vi "Video Stuff v09.vi"() -> ()   [LabVIEW 2009]
uses:
  <vilib>/userDefined/High Color/IMAQdx.ctl
  <vilib>/vision/NI_Vision_Development_Module.lvlib
  <vilib>/vision/driver/NI_Vision_Acquisition_Software.lvlib
panel:
  in  "Y Min":i32=4
  in  "Y Max":i32=22
  in  "X min":i32=4
  in  "X max":i32=22
  in  "Image Type":T1 items=["Grayscale (U8)", "Grayscale (I16)", "Grayscale (SGL)", "Complex (CSG)", "RGB (U32)", "HSL (U32)", "RGB (U64)", "Grayscale (U16)"]
  in  "Desired X Resolution":i32=640
  in  "LineFilterSelect":bool
  out "Hough Intensity Graph":i32[][](graph)
  out "Angle 2":i32
  out "X Intercept 2":i32
  in  "Hough Skip":i32=1
  out "Waypoint":cluster{i32, i32}
  in  "WP_DisplaySize/2":i32
  out "Filter Binary 2":T2(plugin-control)
  in  "Offset scale":dbl=1.51
  in  "Y":i32=1741
  in  "X":i32=777
  out "Real World Coordinates":cluster{"X":sgl, "Y":sgl} {"Y" format="%.2f"; "X" format="%.2f"}
  in  "Interpolation Type":u32(ring)=1 items=["Zero Order", "Bi-Linear", "Quadratic", "Cubic Spline"]
  in  "X Resolution":i32=640
  in  "Filter Select":T3(radio)
  in  "bin 1    bin 2":bool
  in  "Dan    Me":bool=TRUE
  in  "Numeric":i32=21
  out "Occupancy Grid Square Size":dbl
  in  "LIDAR/Wheel Position Offset (in.)":dbl=60.0
  out "\"Obstickles\" y":dbl[](array[numeric])
  out "\"Obstickles\" x":dbl[](array[numeric])
  out "Small":T2(plugin-control)
  in  "Horizontal Resolution of Small Image":i32=50
  out "Super Filter":T2(plugin-control)
  in  "Color Mode":u16(ring) items=["RGB", "HSL", "HSV", "HSI"]
  in  "Blue Range":cluster{"Lower value":i32, "Upper value":i32}={"Lower value"=20, "Upper value"=255}
  in  "Green Range":cluster{"Lower value":i32, "Upper value":i32}={"Lower value"=180, "Upper value"=255}
  in  "Red Range":cluster{"Lower value":i32, "Upper value":i32}={"Lower value"=150, "Upper value"=255}
  in  "stop":bool
  out "trans":T2(plugin-control)
  out "Buffer Number":u32
  out "Live Video":T2(plugin-control)
  in  "Video Modes":i32(listbox)=20
  in  "Camera Name":T4="cam0"
  in  "Calibration File Path":path=path "C:/Documents and Settings/ekolker/My Documents/OGRE/vision/calibrationGridLargeV2.PNG"
  out "Top Image":T2(plugin-control) caption="Calibration Template"
  # "Line Width Paramaters"
  # "Lower:\n   YUV?\n  150, 180, 20\n   RGB?\n  240, 240, 240"
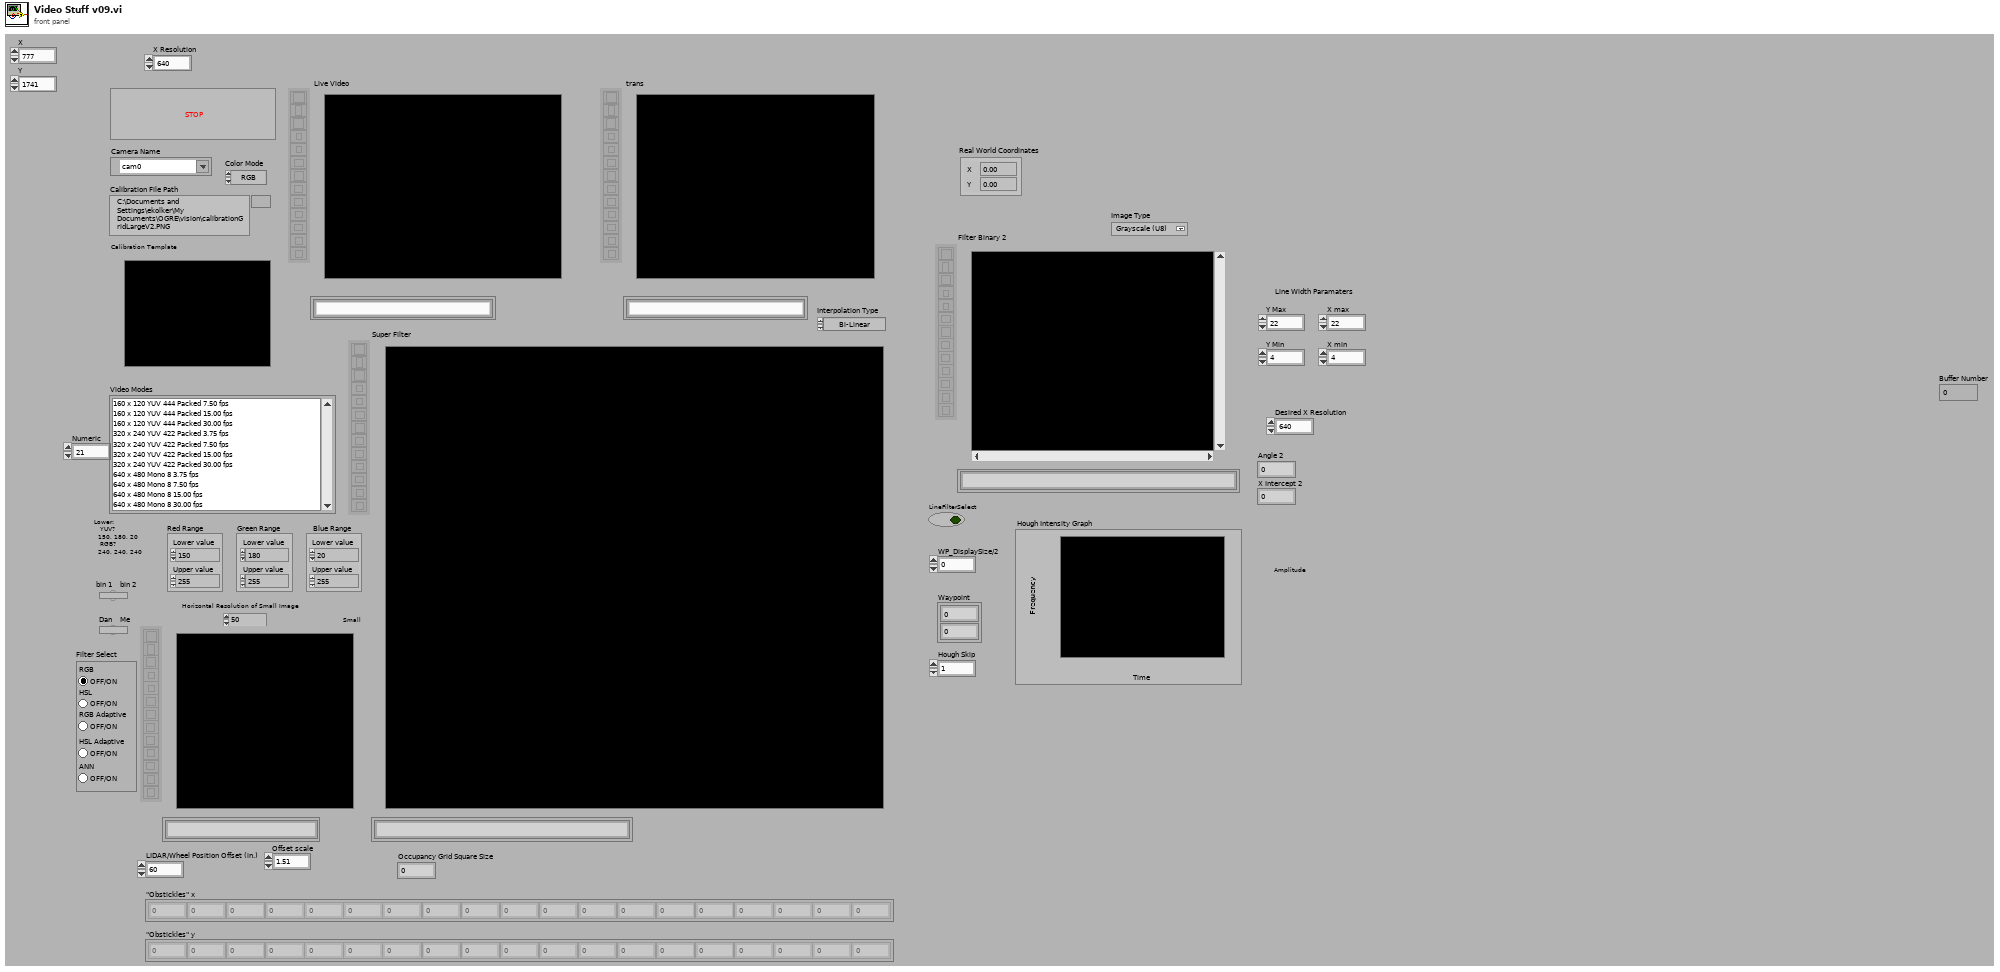
[diagram p1: front panel]
types:
  T1 = typedef "Image Type" = u32
  T2 = typedef "IMAQ Image.ctl" = refnum<image>
  T3 = enum32{"RGB", "HSL", "RGB Adaptive", "HSL Adaptive", "ANN"}
  T4 = typedef "IMAQdx.ctl" = refnum<k21>
  T5 = cluster{"X Step":sgl, "Y Step":sgl, "Unit":u32, "Threshold Range":cluster{"Lower value":sgl, "Upper value":sgl}}
  T6 = cluster{"Distortion":u32, "Corrected Image Scaling":u32, "Corrected Image Learn ROI":u32, "Learn Error Map?":bool, "Learn Correction Table?":bool}
  T7 = cluster{cluster{sgl, sgl}, "Angle Relative to Horizontal (deg)":sgl, "Axis Reference":u32}
  T8 = cluster{"Left":i32, "Top":i32, "Right":i32, "Bottom":i32}
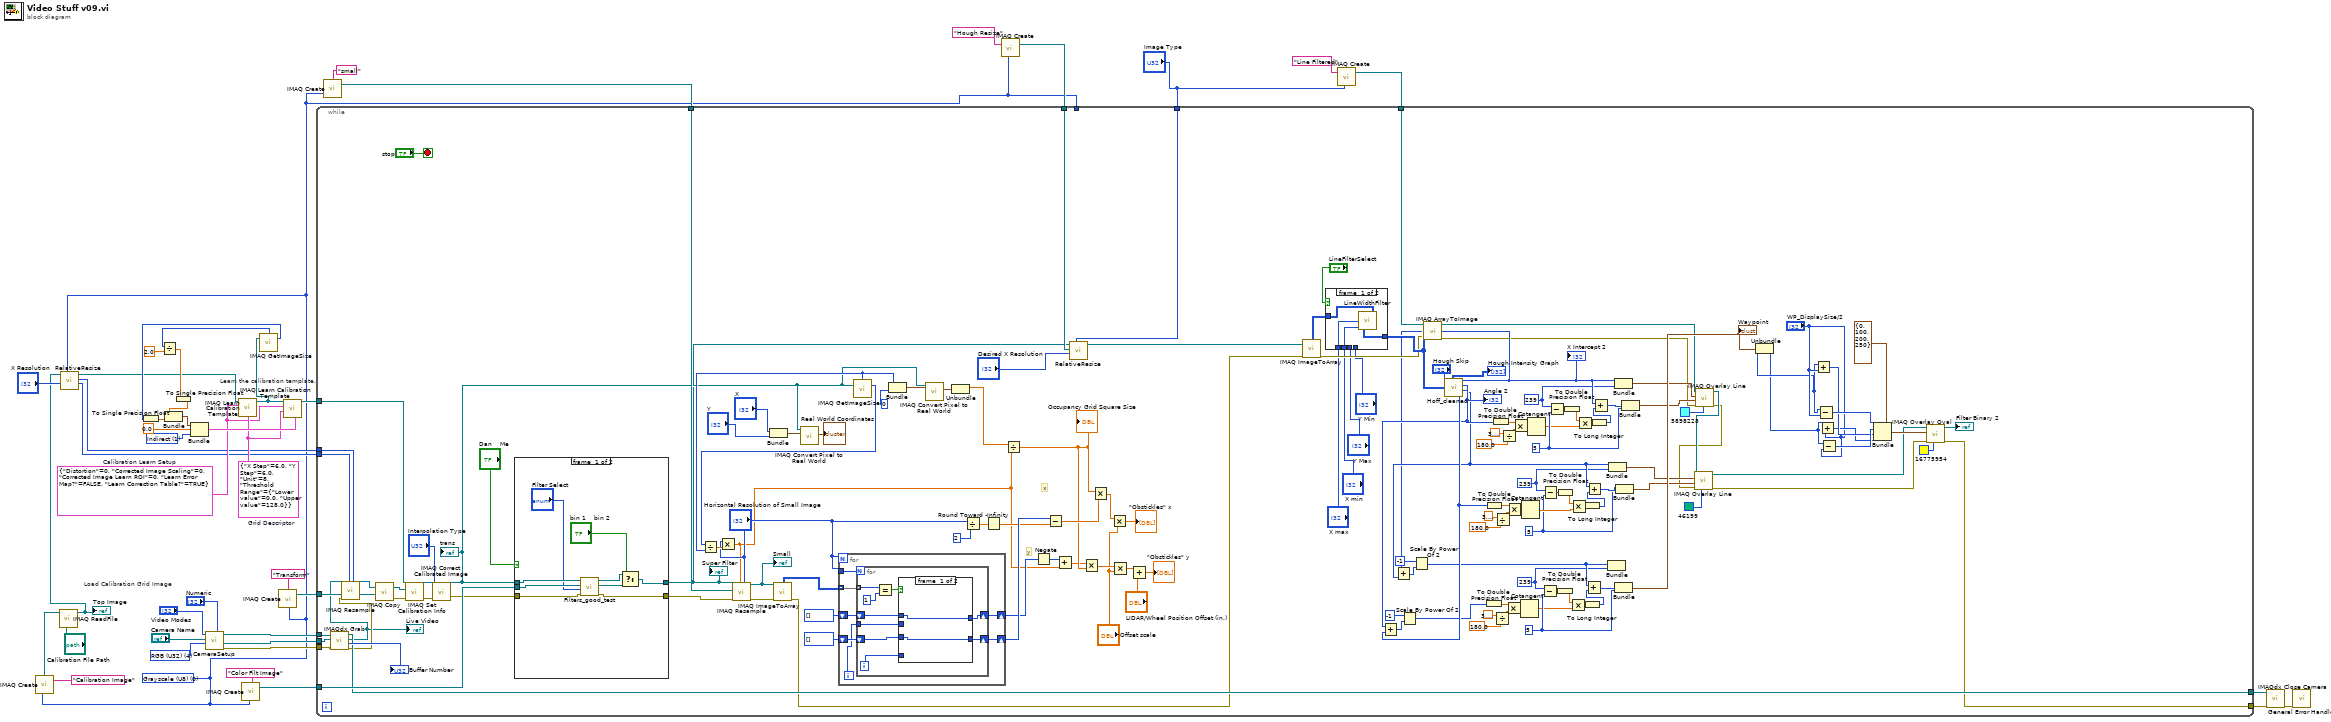
[diagram p0: block diagram]
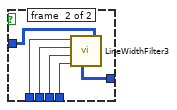
[diagram p2: hidden frame]
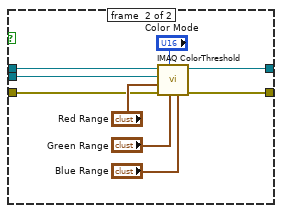
[diagram p3: hidden frame]
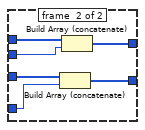
[diagram p4: hidden frame]
diagram:
  w1 = T1 4 items=["Grayscale (U8)", "Grayscale (I16)", "Grayscale (SGL)", "Complex (CSG)", "RGB (U32)", "HSL (U32)", "RGB (U64)", "Grayscale (U16)"] ("Image Type")
  w26 = u32 1 items=["Direct", "Indirect"] ("Axis Reference")
  w3 = T1 0 items=["Grayscale (U8)", "Grayscale (I16)", "Grayscale (SGL)", "Complex (CSG)", "RGB (U32)", "HSL (U32)", "RGB (U64)", "Grayscale (U16)"] ("Image Type")
  w14 = T5 {"X Step"=6.0, "Y Step"=6.0, "Unit"=8, "Threshold Range"={"Lower value"=0.0, "Upper value"=128.0}}  # Grid Descriptor
  w13 = T6 {"Distortion"=0, "Corrected Image Scaling"=0, "Corrected Image Learn ROI"=0, "Learn Error Map?"=FALSE, "Learn Correction Table?"=TRUE}  # Calibration Learn Setup
  # "Load Calibration Grid Image"
  # "Learn the calibration template."
  n1 = call "IMAQ Create"("Image Name"="Calibration Image", "Image Type"=w3) -> ("New Image"=w34:T2)  [unwired: 2 in, 2 out]
  n2 = call "IMAQ ReadFile"("File Path"="Calibration File Path", "Image"=w34) -> ("Image Out"=w8:T2)  [unwired: 3 in, 6 out]
  "Top Image" <- w8
  n3 = call "RelativeResize.vi"("Image Type"=w3, "Desired X Resolution"="X Resolution", "Image"=w8) -> ("Y Resolution"=w6:i32, "X Resolution"=w7:i32, "Image Dst Out"=w9:T2)  [unwired: 3 in, 1 out]
  n4 = call "CameraSetup.vi"("Video Modes"="Video Modes", "Camera Name"="Camera Name", "Image Type"=w1, "Numeric"="Numeric") -> ("Session Out"=w37:T4, "New Image"=w36:T2, "error out"=w35:errorcluster)  [unwired: 2 in]
  n5 = call "IMAQ Learn Calibration Template"("Grid Descriptor"=w14, "Calibration Learn Setup"=w13, "Image"=w9) -> ("Calibrated Image"=w21:T2)  [unwired: 4 in, 4 out]
  n6 = call "IMAQ Create"("Image Name"="Color Filt Image", "Image Type"=w3) -> ("New Image"=w33:T2)  [unwired: 2 in, 2 out]
  n7 = call "IMAQ GetImageSize"("Image"=w21) -> ("Y Resolution"=w18:i32, "X Resolution"=w19:i32)  [unwired: 3 in, 1 out]
  n8 = To Single Precision Float(number=w18) -> (single precision float=w17:sgl)
  n9 = Divide(x=w19, y=2.0) -> (x/y=w16:dbl)
  n10 = To Single Precision Float(number=w16) -> (single precision float=w15:sgl)
  n11 = Bundle(w15, w17) -> (w24:cluster{sgl, sgl})  [unwired: 1 in]
  n12 = Bundle(w24, "Angle Relative to Horizontal (deg)"=sgl 0.0, "Axis Reference"=w26) -> (w22:T7)  [unwired: 1 in]
  n13 = call "IMAQ Create"("Image Name"="Transform", "Image Type"=w3) -> ("New Image"=w38:T2)  [unwired: 2 in, 2 out]
  n14 = call "IMAQ Learn Calibration Template"("Calibration Axis Info"=w22, "Grid Descriptor"=w14, "Calibration Learn Setup"=w13, "Image"=w21) -> ("Calibrated Image"=w23:T2)  [unwired: 3 in, 4 out]
  n15 = call "IMAQ Create"("Image Name"="small", "Image Type"=w3) -> ("New Image"=w31:T2)  [unwired: 2 in, 2 out]
  n16 = call "IMAQ Create"("Image Name"="Hough Resize", "Image Type"=w3) -> ("New Image"=w4:T2)  [unwired: 2 in, 2 out]
  n17 = call "IMAQ Create"("Image Name"="Line Filtered", "Image Type"="Image Type") -> ("New Image"=w11:T2)  [unwired: 2 in, 2 out]
  n18 = while {
    tunnel: w23 -> [w159]
    tunnel: w38 -> [w188]
    tunnel: w37 -> [w187]
    tunnel: w36 -> [w186]
    tunnel: w35 -> [w185]
    tunnel: w33 -> [w181]
    tunnel: w31 -> [w179]
    tunnel: [w177] -> w29
    tunnel: [w120] -> w28
    tunnel: w11 -> [w119]
    tunnel: w7 -> [w59]
    tunnel: w6 -> [w58]
    tunnel: w4 -> [w55]
    tunnel: w3 -> [_]
    tunnel: "Image Type" -> [w54]
    stop <- "stop" stop-if-true
    w104 = 5 ("y")
    w103 = 239 ("y")
    w82 = 5 ("y")
    w83 = 239 ("y")
    w71 = 5 ("y")
    w70 = 239 ("y")
    # "y"
    # "x"
    n19 = call <vilib>:"IMAQdx Grab.vi"("error in"=w185, "Image In"=w186, "Session In"=w187) -> ("error out"=w162:errorcluster, "Buffer Number Out"=→"Buffer Number":u32, "Image Out"=w161:T2, "Session Out"=w177:T4)  [unwired: 1 in, 4 out]
    "Live Video" <- w161
    n20 = call "IMAQ Resample"("X Resolution"=w59, "Y Resolution"=w58, "error in (no error)"=w162, "Image Src"=w161) -> ("Image Dst Out"=w160:T2)  [unwired: 6 in, 1 out]
    n21 = call "IMAQ Copy"("Image Dst"=w188, "Image Src"=w160) -> ("error out"=w189:errorcluster, "Image Dst Out"=w192:T2)  [unwired: 4 in]
    n22 = call "IMAQ Set Calibration Info"("error in (no error)"=w189, "Image Dst"=w192, "Image Src"=w159) -> ("error out"=w190:errorcluster, "Calibrated Image"=w191:T2)  [unwired: 1 in, 6 out]
    n23 = call "IMAQ Correct Calibrated Image"("Interpolation Type"="Interpolation Type", "error in (no error)"=w190, "Image Src"=w191) -> ("error out"=w180:errorcluster, "Corrected Image"=w51:T2)  [unwired: 4 in, 3 out]
    "trans" <- w51
    n24 = case shown="False" "Dan    Me" {
      tunnel: [w211 w217] -> w184
      tunnel: [w208 w216] -> w50
      tunnel: w181 -> [w209 w215]
      tunnel: w180 -> [w212 w214]
      tunnel: w51 -> [w210 w213]
      frame #0 {
        n25 = call "Filters_good_test.vi"("error in"=w212, "Filter Select"="Filter Select", "Filter"=w209, "Input"=w210) -> ("error out"=w211:errorcluster, "Filter Binary"=w207:T2, "Filter Binary 2"=w206:T2)  [unwired: 5 in]
        n26 = Select(t=w206, s="bin 1    bin 2", f=w207) -> (s? t:f=w208:T2)
      }
      frame #1 {
        n27 = call "IMAQ ColorThreshold"("Blue or Luma or Val or Inten Range"="Blue Range", "Green or Sat Range"="Green Range", "Color Mode"="Color Mode", "error in (no error)"=w214, "Red or Hue Range"="Red Range", "Image Dst"=w215, "Image Src"=w213) -> ("error out"=w217:errorcluster, "Image Dst Out"=w216:T2)  [unwired: 3 in]
      }
    }
    "Super Filter" <- w50
    n28 = Bundle("X"="X", "Y"="Y") -> (w155:cluster{"X":i32, "Y":i32})  [unwired: 1 in]
    n29 = call "IMAQ Convert Pixel to Real World"("Pixel Coordinates"=w155, "Calibrated Image"=w51) -> ("Real World Coordinates"=→"Real World Coordinates":cluster{"X":sgl, "Y":sgl})  [unwired: 4 in, 5 out]
    n30 = call "IMAQ GetImageSize"("Image"=w51) -> ("Y Resolution"=w147:i32, "X Resolution"=w146:i32)  [unwired: 3 in, 1 out]
    n31 = Divide(x=w147, y=w146) -> (x/y=w149:dbl)
    n32 = Multiply(x="Horizontal Resolution of Small Image", y=w149) -> (x*y=w140:dbl)
    n33 = call "IMAQ Resample"("X Resolution"="Horizontal Resolution of Small Image", "Y Resolution"=w140, "error in (no error)"=w184, "Image Dst"=w179, "Image Src"=w50) -> ("error out"=w183:errorcluster, "Image Dst Out"=w123:T2)  [unwired: 5 in]
    "Small" <- w123
    n34 = call "IMAQ ImageToArray"("error in (no error)"=w183, "Image"=w123) -> ("error out"=w121:errorcluster, "Image Pixels (U8)"=w174:u8[][])  [unwired: 2 in, 3 out]
    n35 = for {
      N: "Horizontal Resolution of Small Image" -> [_]
      tunnel: "Horizontal Resolution of Small Image" -> [w228]
      tunnel: w174 -> [w227] mode=indexing
      shift-right: [w226] -> w173
      shift-left: i32[] [] -> [w225]
      shift-right: [w223] -> w166
      shift-left: i32[] [] -> [w222]
      i -> [w224]
      n36 = for {
        N: w228 -> [_]
        tunnel: w227 -> [w237] mode=indexing
        shift-right: [w233] -> w226
        shift-left: w225 -> [w232]
        tunnel: w224 -> [w231]
        shift-right: [w230] -> w223
        shift-left: w222 -> [w229]
        i -> [w235]
        n37 = Equal?(x=w237, y=u8 1) -> (x = y?=w234:bool)
        n38 = case shown="False" w234 {
          tunnel: w235 -> [_ w245]
          tunnel: [w238 w244] -> w233
          tunnel: w232 -> [w238 w243]
          tunnel: w231 -> [_ w242]
          tunnel: [w239 w241] -> w230
          tunnel: w229 -> [w239 w240]
          frame #0 {
          }
          frame #1 {
            n39 = Build Array (concatenate)(w243, w245) -> (w244:i32[])
            n40 = Build Array (concatenate)(w240, w242) -> (w241:i32[])
          }
        }
      }
    }
    n41 = Bundle("X Resolution"=w146, 0) -> (w157:cluster{"X Resolution":i32, i32})  [unwired: 1 in]
    n42 = call "IMAQ Convert Pixel to Real World"("Pixel Coordinates"=w157, "Calibrated Image"=w51) -> ("Real World Coordinates"=w151:cluster{"X":sgl, "Y":sgl})  [unwired: 4 in, 5 out]
    n43 = Unbundle(w151) -> ("X"=w150:sgl)  [unwired: 1 out]
    n44 = Divide(x="Horizontal Resolution of Small Image", y=2) -> (x/y=w165:dbl)
    n45 = Round Toward -Infinity(1:w165) -> (0:w164:dbl)
    n46 = Divide(x=w150, y=w140) -> (x/y=w171:dbl)
    "Occupancy Grid Square Size" <- w171
    n47 = Negate(x=w166) -> (-x=w167:i32[])
    n48 = Subtract(x=w173, y=w164) -> (x-y=w172:dbl[])
    n49 = Add(x=w167, y=w140) -> (x+y=w170:dbl[])
    n50 = call "RelativeResize.vi"("Image Type"=w54, "Desired X Resolution"="Desired X Resolution", "Image Dst"=w55, "Image"=w50) -> ("Image Dst Out"=w57:T2)  [unwired: 2 in, 3 out]
    n51 = Multiply(x=w170, y=w171) -> (x*y=w145:dbl[])
    n52 = Multiply(x=w171, y=w172) -> (x*y=w143:dbl[])
    n53 = Multiply(x=w143, y="Offset scale") -> (x*y=→"\"Obstickles\" x":dbl[])
    n54 = Multiply(x=w145, y="Offset scale") -> (x*y=w144:dbl[])
    n55 = Add(x=w144, y="LIDAR/Wheel Position Offset (in.)") -> (x+y=→"\"Obstickles\" y":dbl[])
    n56 = call "IMAQ ImageToArray"("error in (no error)"=w121, "Image"=w57) -> ("error out"=w122:errorcluster, "Image Pixels (U8)"=w124:u8[][])  [unwired: 2 in, 3 out]
    n57 = case shown="False" "LineFilterSelect" {
      tunnel: w124 -> [w195 w202]
      tunnel: [w197 w203] -> w127
      tunnel: "X max" -> [w196 w201]
      tunnel: "X min" -> [w194 w200]
      tunnel: "Y Max" -> [_ w199]
      tunnel: "Y Min" -> [_ w198]
      frame #0 {
        n58 = call "LineWidthFilter.vi"("Image Pixels (U8) 2"=w195, "X Min"=w194, "X max"=w196) -> ("Image Pixels (U8)"=w197:u8[][])
      }
      frame #1 {
        n59 = call "LineWidthFilter3.vi"("X max"=w201, "X min"=w200, "Y Max"=w199, "Y Min"=w198, "Image Pixels (U8) 2"=w202) -> ("Image Pixels (U8)"=w203:u8[][])
      }
    }
    n60 = call "IMAQ ArrayToImage"("error in (no error)"=w122, "Image Pixels (U8)"=w127, "Image"=w119) -> ("error out"=w60:errorcluster, "Image Out"=w53:T2)  [unwired: 7 in]
    n61 = call "Hoff_cleaned.vi"("Skip-1"="Hough Skip", "Image Pixels (U8)"=w127) -> ("3 times averaged"=→"Hough Intensity Graph":i32[][], "X Intercept"=w115:i32, "Angle"=w117:i32, "X Intercept 2"=w116:i32, "Angle 2"=w118:i32)  [unwired: 2 in]
    "Angle 2" <- w117
    "X Intercept 2" <- w115
    n62 = Add(x=w117, y=w118) -> (x+y=w114:i32)
    n63 = Add(x=w115, y=w116) -> (x+y=w113:i32)
    n64 = Scale By Power Of 2(n=i16 -1, x=w114) -> (x*2^n=w110:i32)
    n65 = Scale By Power Of 2(n=i16 -1, x=w113) -> (x*2^n=w112:i32)
    n66 = To Double Precision Float(number=w110) -> (double precision float=w98:dbl)
    n67 = To Double Precision Float(number=w118) -> (double precision float=w88:dbl)
    n68 = To Double Precision Float(number=w117) -> (double precision float=w65:dbl)
    n69 = Divide(x=3.141592653589793, y=180.0) -> (x/y=w99:dbl)
    n70 = Divide(x=3.141592653589793, y=180.0) -> (x/y=w87:dbl)
    n71 = Divide(x=3.141592653589793, y=180.0) -> (x/y=w66:dbl)
    n72 = Multiply(x=w98, y=w99) -> (x*y=w100:dbl)
    n73 = Multiply(x=w88, y=w87) -> (x*y=w86:dbl)
    n74 = Multiply(x=w65, y=w66) -> (x*y=w67:dbl)
    n75 = Cotangent(1:w100) -> (0:w101:dbl)
    n76 = Cotangent(1:w86) -> (0:w85:dbl)
    n77 = Cotangent(1:w67) -> (0:w68:dbl)
    n78 = Subtract(x=w103, y=w104) -> (x-y=w105:i32)
    n79 = Subtract(x=w83, y=w82) -> (x-y=w81:i32)
    n80 = Subtract(x=w70, y=w71) -> (x-y=w74:i32)
    n81 = To Double Precision Float(number=w105) -> (double precision float=w106:dbl)
    n82 = To Double Precision Float(number=w81) -> (double precision float=w80:dbl)
    n83 = To Double Precision Float(number=w74) -> (double precision float=w75:dbl)
    n84 = Multiply(x=w106, y=w101) -> (x*y=w107:dbl)
    n85 = Multiply(x=w80, y=w85) -> (x*y=w79:dbl)
    n86 = Multiply(x=w75, y=w68) -> (x*y=w76:dbl)
    n87 = To Long Integer(number=w107) -> (32bit integer=w108:i32)
    n88 = To Long Integer(number=w79) -> (32bit integer=w78:i32)
    n89 = Add(x=w112, y=w108) -> (x+y=w102:i32)
    n90 = Add(x=w116, y=w78) -> (x+y=w84:i32)
    n91 = To Long Integer(number=w76) -> (32bit integer=w77:i32)
    n92 = Add(x=w115, y=w77) -> (x+y=w69:i32)
    n93 = Bundle(w112, "y"=w103) -> ()  [unwired: 1 in, 1 out]
    n94 = Bundle("X Intercept 2"=w116, "y"=w83) -> (w93:cluster{"X Intercept 2":i32, "y":i32})  [unwired: 1 in]
    n95 = Bundle("X Intercept"=w115, "y"=w70) -> (w72:cluster{"X Intercept":i32, "y":i32})  [unwired: 1 in]
    n96 = Bundle(w102, "y"=w104) -> (w128:cluster{i32, "y":i32})  [unwired: 1 in]
    "Waypoint" <- w128
    n97 = Bundle(w84, "y"=w82) -> (w94:cluster{i32, "y":i32})  [unwired: 1 in]
    n98 = Bundle(w69, "y"=w71) -> (w73:cluster{i32, "y":i32})  [unwired: 1 in]
    n99 = call "IMAQ Overlay Line"("Color"=u32 5898228, "error in (no error)"=w60, "End Point"=w73, "Start Point"=w72, "Image"=w53) -> ("error out"=w45:errorcluster, "Image Out"=w95:T2)  [unwired: 5 in]
    n100 = call "IMAQ Overlay Line"("Color"=u32 46199, "error in (no error)"=w45, "End Point"=w94, "Start Point"=w93, "Image"=w95) -> ("error out"=w125:errorcluster, "Image Out"=w131:T2)  [unwired: 5 in]
    n101 = Unbundle(w128) -> (w130:i32, "y"=w129:i32)
    n102 = Add(x=w130, y="WP_DisplaySize/2") -> (x+y=w136:i32)
    n103 = Subtract(x=w130, y="WP_DisplaySize/2") -> (x-y=w138:i32)
    n104 = Add(x=w129, y="WP_DisplaySize/2") -> (x+y=w135:i32)
    n105 = Subtract(x=w129, y="WP_DisplaySize/2") -> (x-y=w137:i32)
    n106 = Bundle(cluster=T8 {"Left"=0, "Top"=100, "Right"=200, "Bottom"=250} ("Bounding Rectangle"), "Left"=w138, "Top"=w137, "Right"=w136, "Bottom"=w135) -> (w134:T8)
    n107 = call "IMAQ Overlay Oval"("Color"=u32 16775954, "error in (no error)"=w125, "Bounding Rectangle"=w134, "Image"=w131) -> ("error out"=w120:errorcluster, "Image Out"=→"Filter Binary 2":T2)  [unwired: 6 in]
  }
  n108 = call <vilib>:"IMAQdx Close Camera.vi"("error in"=w28, "Session In"=w29) -> ("error out"=w30:errorcluster)  [unwired: 9 out]
  n109 = call <vilib>:"General Error Handler.vi"("error in (no error)"=w30) -> ()  [unwired: 1 in, 14 out]
